vi "数值+1与布尔数组进位位映射.vi"(11 "U8整型":u8) -> (3 "进位位":i32)   [LabVIEW 2017]
panel:
  out "加一后":bool[](array[boolean])
  out "原数":bool[](array[boolean])
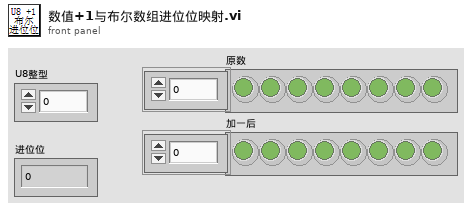
[diagram p1: front panel]
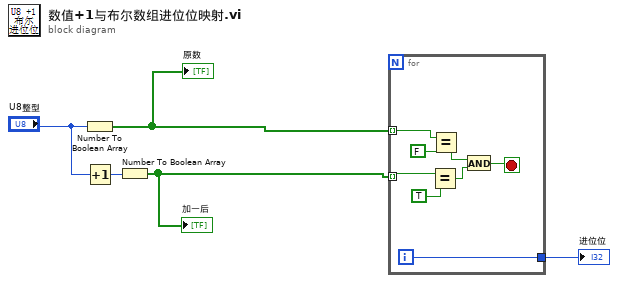
[diagram p0: block diagram]
diagram:
  n1 = Number To Boolean Array(number="U8整型") -> (Boolean array=w2:bool[])
  "原数" <- w2
  n2 = Increment(x="U8整型") -> (x+1=w4:u8)
  n3 = Number To Boolean Array(number=w4) -> (Boolean array=w1:bool[])
  "加一后" <- w1
  n4 = for {
    tunnel: w2 -> [w12] mode=indexing
    tunnel: w1 -> [w11] mode=indexing
    tunnel: [w7] -> w3
    i -> [w7]
    stop <- w8 stop-if-true
    n5 = Equal?(x=w11, y=TRUE) -> (x = y?=w10:bool)
    n6 = Equal?(x=w12, y=FALSE) -> (x = y?=w9:bool)
    n7 = And(x=w9, y=w10) -> (x .and. y?=w8:bool)
  }
  "进位位" <- w3
